vi "endLaserComms.vi"(0 "outputLasers":T1(array[cluster])) -> ()   [LabVIEW 2015]
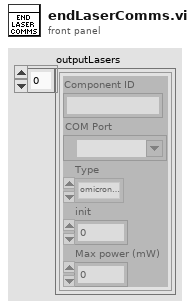
[diagram p1: front panel]
types:
  T1 = cluster{"Component ID":string, "COM Port":refnum<visa-resource-name>, "Type ":enum16{"omicronLuxX", "coherentObis"}, "init":i16, "Max power (mW)":dbl}[]
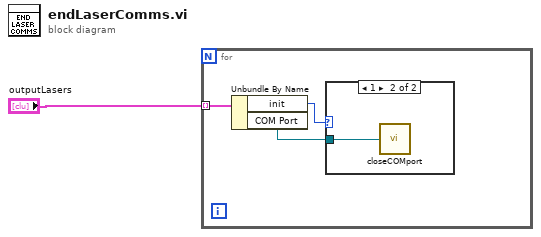
[diagram p0: block diagram]
diagram:
  n1 = for {
    tunnel: "outputLasers" -> [w4] mode=indexing
    n2 = Unbundle By Name(w4) -> ("init"=w3:i16, "COM Port"=w2:refnum<visa-resource-name>)
    n3 = case shown="1" w3 {
      tunnel: w2 -> [_ w5]
      frame 0, Default {
      }
      frame 1 {
        n4 = call "closeCOMport.vi"("COM port"=w5) -> ()
      }
    }
  }
